vi "ControlsPositions.vi"(6 "Ref?":bool, 8 "error in (no error)":errorcluster, 9 "Boolean":bool=TRUE, 11 "Referencia":T1) -> (0 "error out":errorcluster)   [LabVIEW 2021]
uses:
  Typedefs/Referencias.ctl
  Typedefs/Axis.ctl
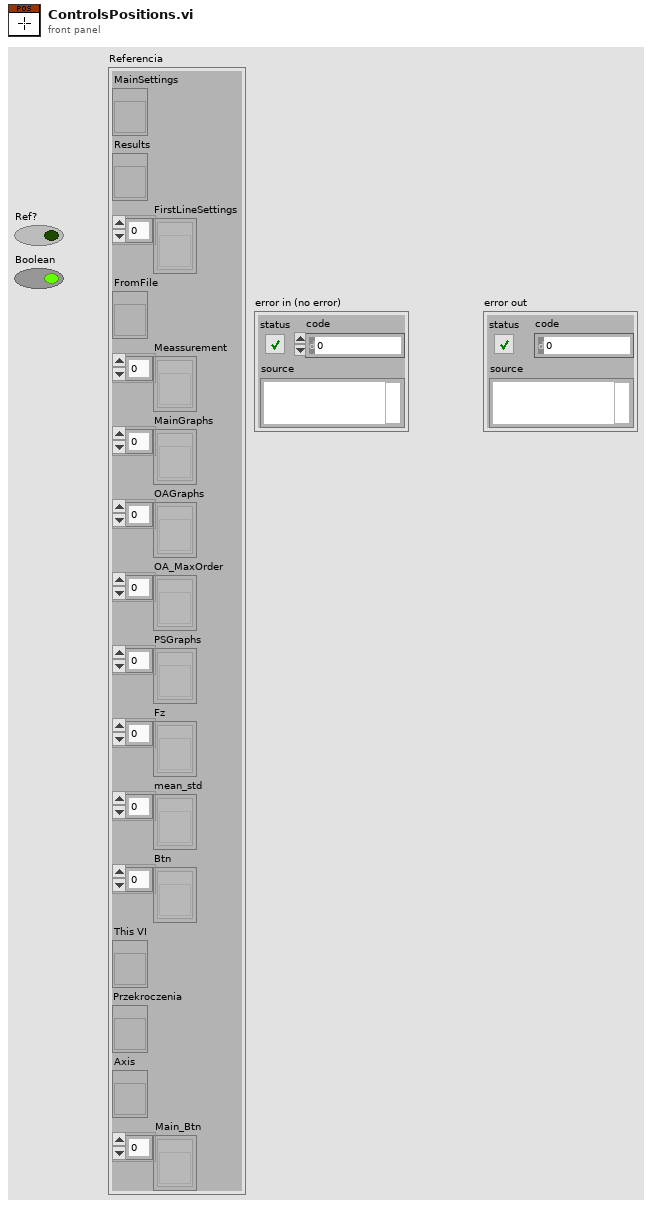
[diagram p1: front panel]
types:
  T1 = typedef "Referencias.ctl" = cluster{"MainSettings":refnum<vi>, "Results":refnum<vi>, "FirstLineSettings":refnum<vi>[], "FromFile":refnum<vi>, "Meassurement":refnum<vi>[], "MainGraphs":refnum<vi>[], "OAGraphs":refnum<vi>[], "OA_MaxOrder":refnum<vi>[], "PSGraphs":refnum<vi>[], "Fz":refnum<vi>[], "mean_std":refnum<vi>[], "Btn":refnum<vi>[], "This VI":refnum<vi>, "Przekroczenia":refnum<vi>, "Axis":refnum<vi>, "Main_Btn":refnum<vi>[]}
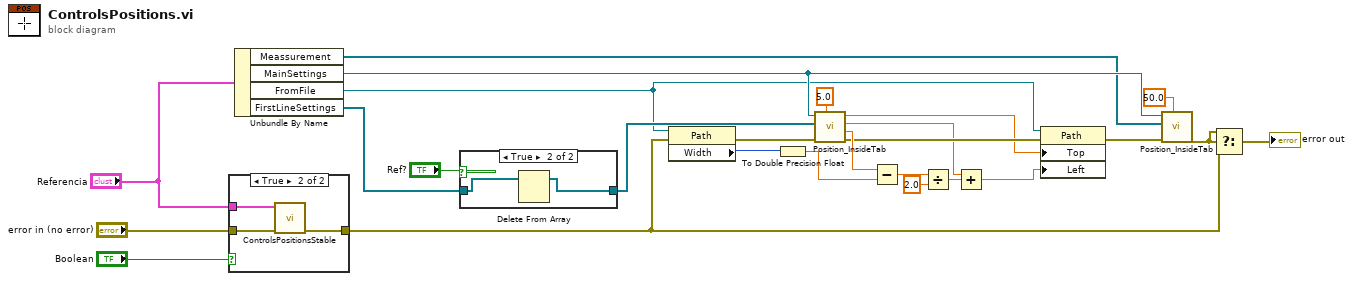
[diagram p0: block diagram]
diagram:
  n1 = case shown="True" "Boolean" {
    tunnel: "Referencia" -> [_ w30]
    tunnel: "error in (no error)" -> [w27 w29]
    tunnel: [w27 w28] -> w1
    frame False {
    }
    frame True {
      n2 = call "ControlsPositionsStable.vi"("error in (no error)"=w29, "Referencia"=w30) -> ("error out"=w28:errorcluster)  [unwired: 9 in]
    }
  }
  n3 = Unbundle By Name("Referencia") -> ("Meassurement"=w8:refnum<vi>[], "MainSettings"=w9:refnum<vi>, "FromFile"=w7:refnum<vi>, "FirstLineSettings"=w10:refnum<vi>[])
  n4 = case shown="True" "Ref?" {
    tunnel: w10 -> [w31 w33]
    tunnel: [w31 w32] -> w11
    frame False {
    }
    frame True {
      n5 = Delete From Array(array=w33) -> (array with subset deleted=w32:refnum<vi>[])  [unwired: 2 in, 1 out]
    }
  }
  n6 = property class="Path"(reference=w7, error in=w1) -> (error out=w25:errorcluster, "Width"=w20:u32)  [unwired: 1 out]
  n7 = To Double Precision Float(number=w20) -> (double precision float=w24:dbl)
  n8 = call "Position_InsideTab.vi"("Top"=5.0, "error in (no error)"=w25, "FirstLineSettings"=w11, "TabControl in"=w9) -> ("error out"=w18:errorcluster, "Width"=w19:dbl, "Left"=w17:dbl, "Top"=w14:dbl)  [unwired: 4 in]
  n9 = Subtract(x=w19, y=w24) -> (x-y=w23:dbl)
  n10 = Divide(x=w23, y=2.0) -> (x/y=w21:dbl)
  n11 = Add(x=w17, y=w21) -> (x+y=w16:dbl)
  n12 = property class="Path"(reference=w7, error in=w18, "Top"=w14, "Left"=w16) -> (error out=w15:errorcluster)  [unwired: 1 out]
  n13 = call "Position_InsideTab.vi"("Top"=50.0, "error in (no error)"=w15, "FirstLineSettings"=w8, "TabControl in"=w9) -> ("error out"=w5:errorcluster)  [unwired: 4 in, 3 out]
  n14 = Select(t=w5, s=w5, f=w1) -> (s? t:f=→"error out":errorcluster)
